vi "波形发生器模拟输出.vi"() -> ()   [LabVIEW 2017]
uses:
  <vilib>/DAQmx/write.llb/DAQmx Write (Analog Wfm 1Chan NSamp).vi
  <vilib>/DAQmx/create/channels.llb/DAQmx Create Channel (AO-Voltage-Basic).vi
  <vilib>/DAQmx/configure/timing.llb/DAQmx Timing (Sample Clock).vi
  <vilib>/DAQmx/miscellaneous.llb/DAQmx Fill In Error Info.vi
  <resource>/objmgr/daqmx.rc
panel:
  out "采集卡的采样率":dbl
  in  "Fs":dbl=1000.0 caption="采样率" format="%.2p"
  in  "#s":dbl=1000.0 caption="样本数"
  in  "噪声选择":i8(slide)
  out "最小值":dbl format="%#_3g"
  out "最大值":dbl format="%#_3g"
  out "频率":dbl
  in  "自定义波形":cluster{"输入坐标":bool, "手绘":bool, "输入公式":bool}
  in  "波形选择\n选择":bool
  in  "标准波形":i8(slide) scale=0.0..3.0
  out "自定义波形指示灯":bool
  out "标准波形指示灯":bool
  in  "相位":dbl
  in  "幅值":dbl
  in  "频率":dbl
  in  "停止":bool
  in  "噪声幅值":dbl=1.0 format="%.2p"
  in  "占空比":dbl=50.0 caption="占空比(%)" format="%0.2f"
  out "波形图":waveform(dbl)(graph)
  # "函 数 发 生 器"
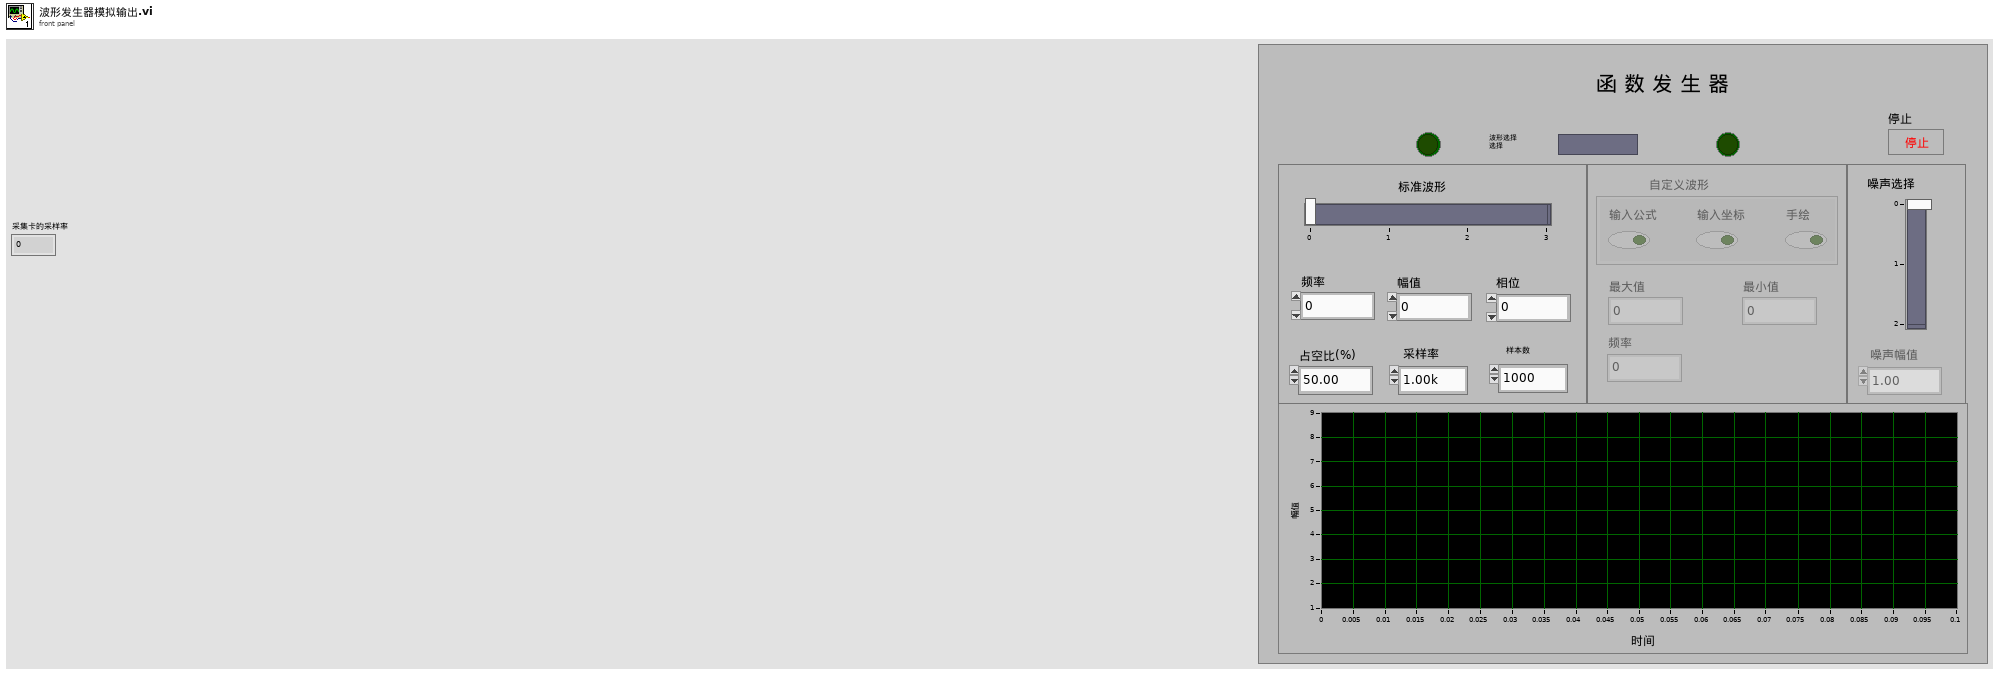
[diagram p1: front panel]
types:
  T1 = enum8{"Enabled", "Disabled", "Disabled and Grayed Out"}
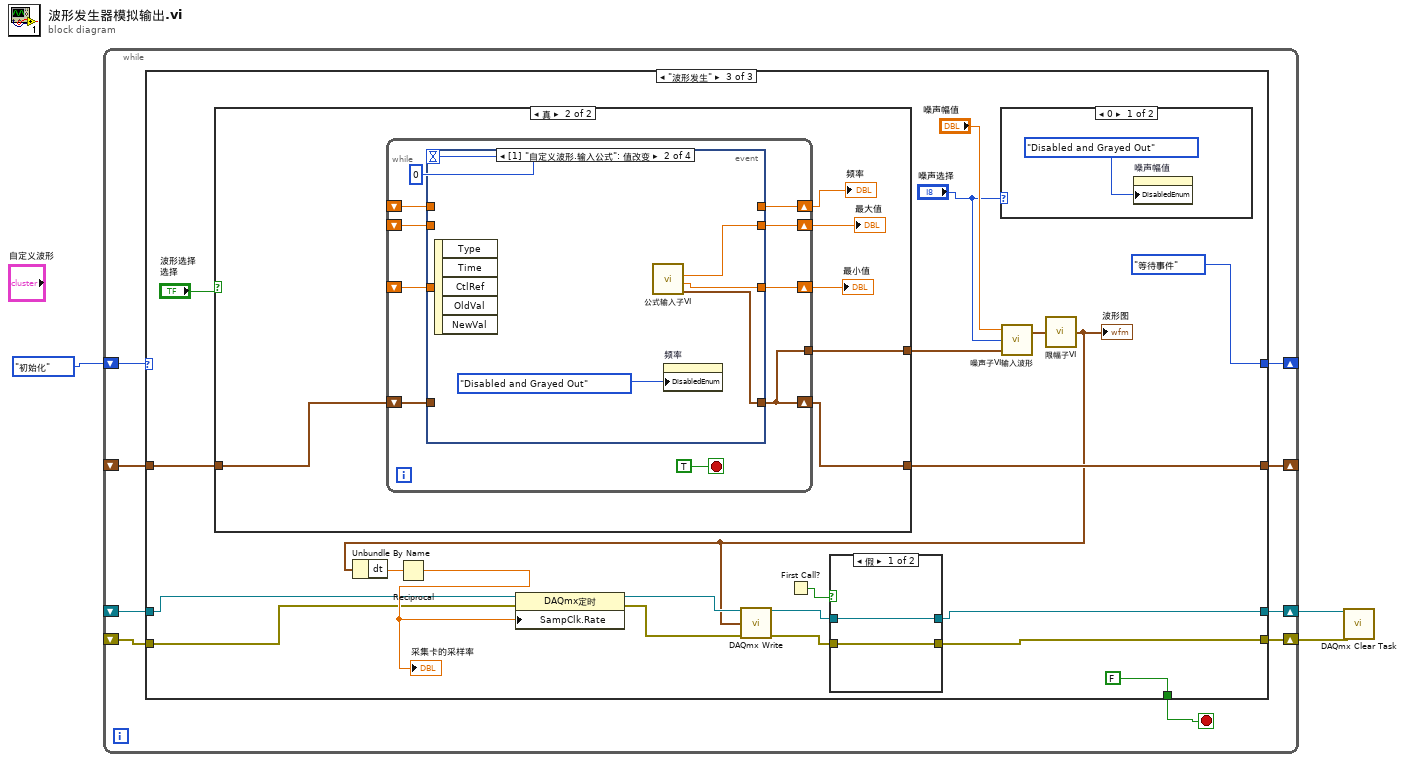
[diagram p0: block diagram]
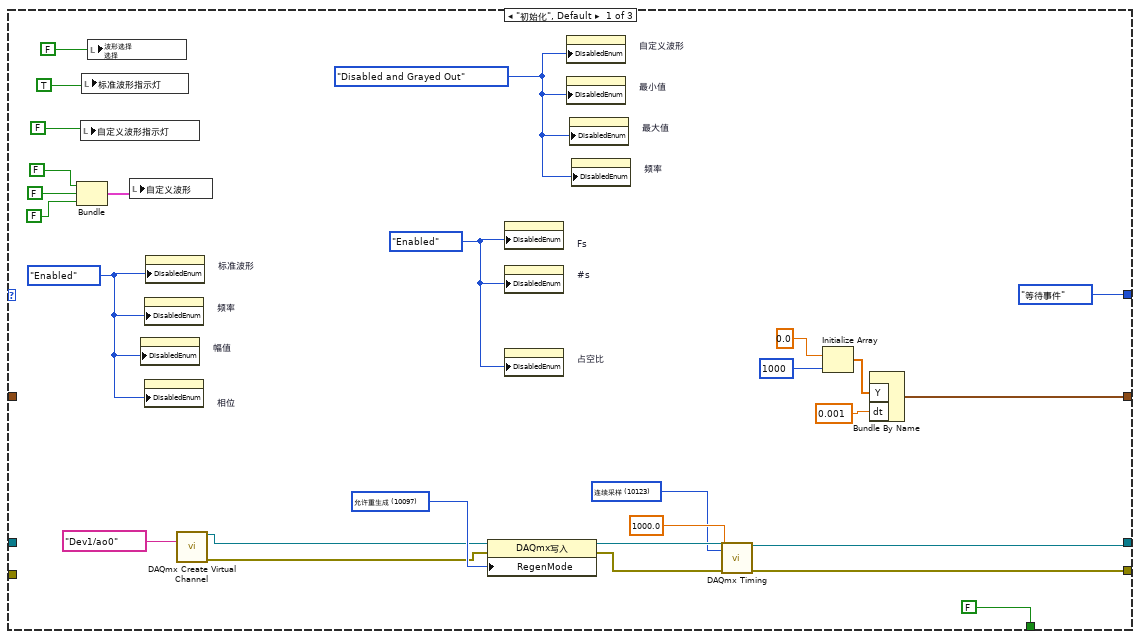
[diagram p2: hidden frame]
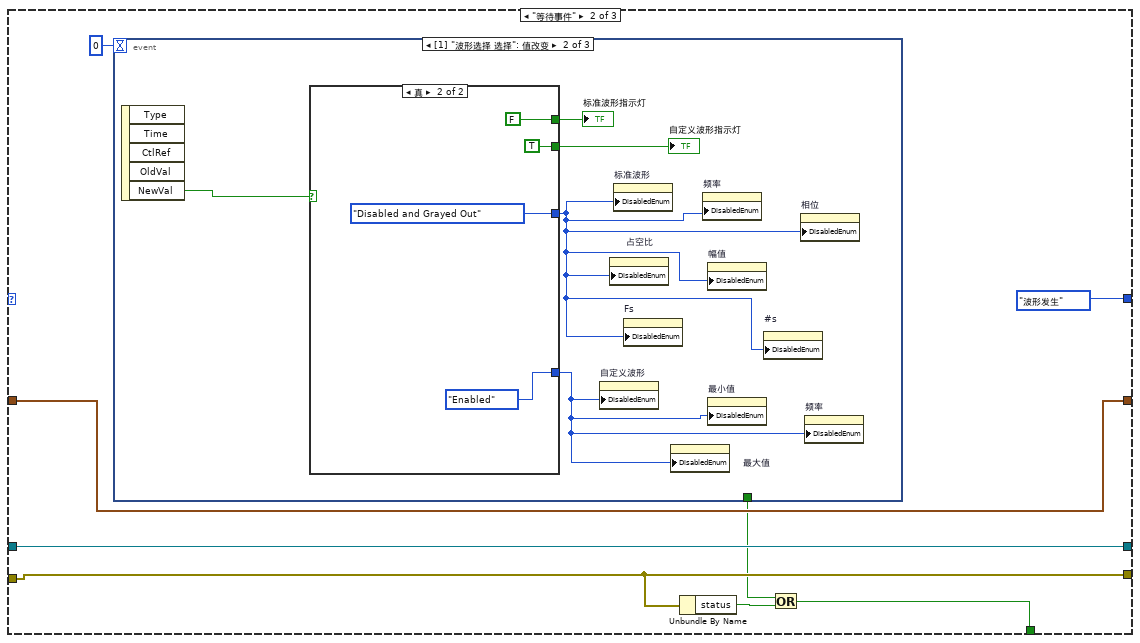
[diagram p3: hidden frame]
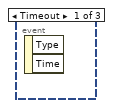
[diagram p4: hidden frame]
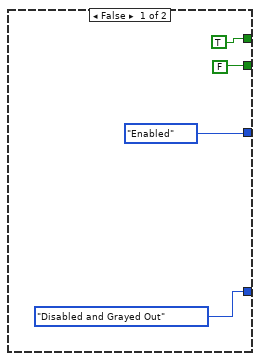
[diagram p5: hidden frame]
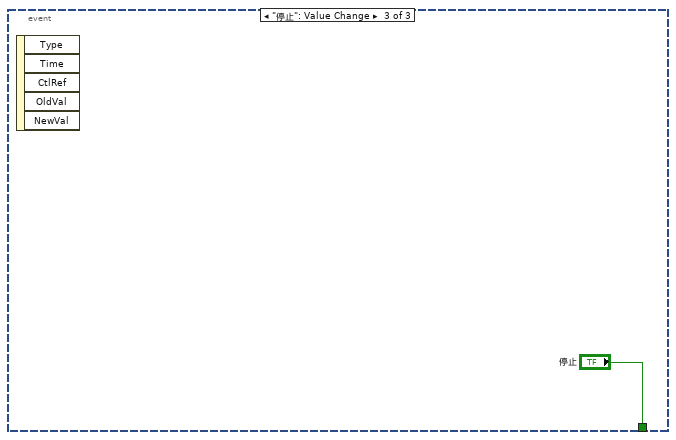
[diagram p6: hidden frame]
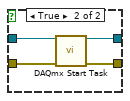
[diagram p7: hidden frame]
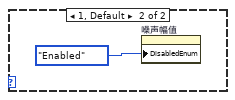
[diagram p8: hidden frame]
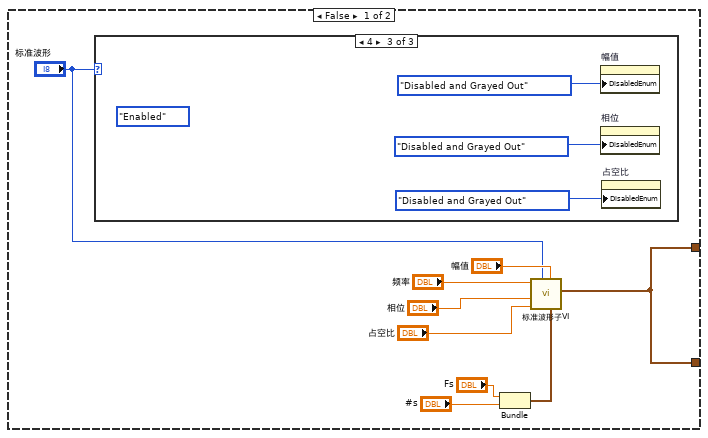
[diagram p9: hidden frame]
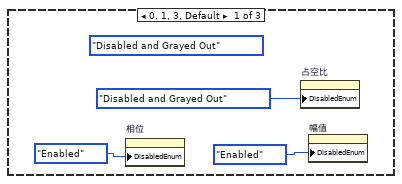
[diagram p10: hidden frame]
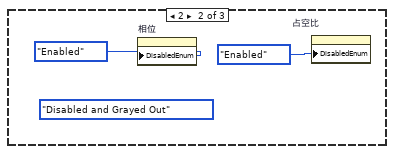
[diagram p11: hidden frame]
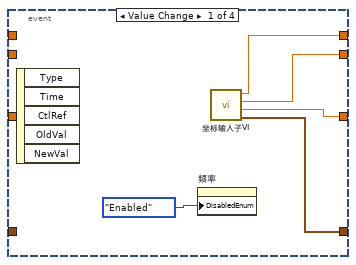
[diagram p12: hidden frame]
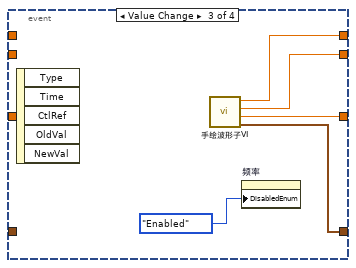
[diagram p13: hidden frame]
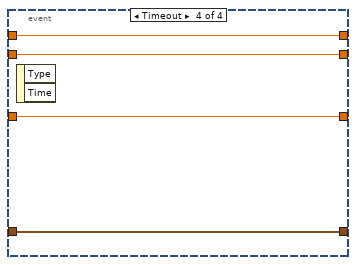
[diagram p14: hidden frame]
diagram:
  n1 = while {
    shift-right: [w11] -> _
    shift-left: enum16{"初始化", "等待事件", "波形发生", "停止"}."初始化" -> [w12]
    shift-right: [w9] -> _
    shift-left: _ -> [w10]
    shift-right: [w6] -> w2
    shift-left: _ -> [w8]
    shift-right: [w5] -> w1
    shift-left: _ -> [w7]
    stop <- w4 stop-if-true
    n2 = case shown="\"波形发生\"" w12 {
      tunnel: [enum16{"初始化", "等待事件", "波形发生", "停止"}."等待事件" enum16{"初始化", "等待事件", "波形发生", "停止"}."波形发生" enum16{"初始化", "等待事件", "波形发生"}."等待事件"] -> w11
      tunnel: w10 -> [_ w47 w76]
      tunnel: [w14 w47 w75] -> w9
      tunnel: w8 -> [_ w46 w66]
      tunnel: w7 -> [_ w44 w65]
      tunnel: [w24 w46 w64] -> w6
      tunnel: [w23 w44 w63] -> w5
      tunnel: [FALSE ("status") w41 FALSE ("status")] -> w4
      frame "初始化", Default {
        w29 = 10097 items=["允许重生成"=10097, "不允许重生成"=10158] ("RegenMode")
        w25 = 10123 items=["有限采样"=10178, "连续采样"=10123, "硬件定时单点"=12522] ("sample mode")
        w31 = T1."Enabled" ("禁用")
        w32 = T1."Enabled" ("禁用")
        w30 = T1."Disabled and Grayed Out" ("禁用")
        n3 = Bundle(FALSE, FALSE, FALSE) -> (w33:cluster{bool, bool, bool})  [unwired: 1 in]
        n4 = local write "自定义波形指示灯"(FALSE ("自定义波形")) -> ()
        n5 = local write "标准波形指示灯"(TRUE ("标准波形")) -> ()
        n6 = local write "波形选择\n选择"(FALSE ("波形选择")) -> ()
        n7 = local write "自定义波形"(w33) -> ()
        n8 = property on="幅值" class="DigNum (严格)"("DisabledEnum"=w32) -> ()  [unwired: 2 in, 2 out]
        n9 = property on="频率" class="DigNum (严格)"("DisabledEnum"=w32) -> ()  [unwired: 2 in, 2 out]
        n10 = property on="相位" class="DigNum (严格)"("DisabledEnum"=w32) -> ()  [unwired: 2 in, 2 out]
        n11 = property on="标准波形" class="Slide (严格)"("DisabledEnum"=w32) -> ()  [unwired: 2 in, 2 out]
        n12 = call-poly <vilib>:"DAQmx Create Virtual Channel.vi"("physical channels"=tag "Dev1/ao0") -> ("task out"=w21:refnum<k21>, "error out"=w20:errorcluster)  [unwired: 13 in]
        n13 = property class="DAQmx写入"(reference=w21, error in=w20, "RegenMode"=w29) -> (reference out=w27:refnum<k21>, error out=w28:errorcluster)
        n14 = property on="Fs" class="DigNum (严格)"("DisabledEnum"=w31) -> ()  [unwired: 2 in, 2 out]
        n15 = property on="#s" class="DigNum (严格)"("DisabledEnum"=w31) -> ()  [unwired: 2 in, 2 out]
        n16 = property on="占空比" class="DigNum (严格)"("DisabledEnum"=w31) -> ()  [unwired: 2 in, 2 out]
        n17 = property on="自定义波形" class="Clust (严格)"("DisabledEnum"=w30) -> ()  [unwired: 2 in, 2 out]
        n18 = property on="最小值" class="DigNum (严格)"("DisabledEnum"=w30) -> ()  [unwired: 2 in, 2 out]
        n19 = property on="最大值" class="DigNum (严格)"("DisabledEnum"=w30) -> ()  [unwired: 2 in, 2 out]
        n20 = property on="频率" class="DigNum (严格)"("DisabledEnum"=w30) -> ()  [unwired: 2 in, 2 out]
        n21 = call-poly <vilib>:"DAQmx Timing.vi"("task/channels in"=w27, "sample mode"=w25, "rate"=1000.0, "error in"=w28) -> ("task out"=w24:refnum<k21>, "error out"=w23:errorcluster)  [unwired: 10 in]
        n22 = Initialize Array(0.0 ("元素"), 1000 ("维数大小")) -> (w17:dbl[])
        n23 = Bundle By Name("Y"=w17, "dt"=0.001) -> (w14:waveform(dbl))  [unwired: 1 in]
      }
      frame "等待事件" {
        n24 = event shown="[1] \"波形选择 选择\": 值改变" {
          selector: _ -> [_ _ _]
          dyn-events: _ -> [_ _ _]
          timeout: 0 -> [_ _ _]
          tunnel: [_ _ "停止"] -> w43
          event Timeout {
            n25 = event-data() -> ()  [unwired: 1 in, 2 out]
          }
          event "波形选择\n选择": Value Change {
            n26 = event-data() -> ("NewVal"=w50:bool)  [unwired: 1 in, 4 out]
            n27 = case shown="真" w50 {
              tunnel: [TRUE FALSE] -> w52
              tunnel: [FALSE TRUE] -> w51
              tunnel: [T1."Enabled" ("禁用") T1."Disabled and Grayed Out" ("禁用")] -> w49
              tunnel: [T1."Disabled and Grayed Out" ("禁用") T1."Enabled" ("禁用")] -> w48
              frame False {
              }
              frame True {
              }
            }
            "标准波形指示灯" <- w52
            "自定义波形指示灯" <- w51
            n28 = property on="自定义波形" class="Clust (严格)"("DisabledEnum"=w48) -> ()  [unwired: 2 in, 2 out]
            n29 = property on="占空比" class="DigNum (严格)"("DisabledEnum"=w49) -> ()  [unwired: 2 in, 2 out]
            n30 = property on="标准波形" class="Slide (严格)"("DisabledEnum"=w49) -> ()  [unwired: 2 in, 2 out]
            n31 = property on="Fs" class="DigNum (严格)"("DisabledEnum"=w49) -> ()  [unwired: 2 in, 2 out]
            n32 = property on="最大值" class="DigNum (严格)"("DisabledEnum"=w48) -> ()  [unwired: 2 in, 2 out]
            n33 = property on="频率" class="DigNum (严格)"("DisabledEnum"=w49) -> ()  [unwired: 2 in, 2 out]
            n34 = property on="幅值" class="DigNum (严格)"("DisabledEnum"=w49) -> ()  [unwired: 2 in, 2 out]
            n35 = property on="最小值" class="DigNum (严格)"("DisabledEnum"=w48) -> ()  [unwired: 2 in, 2 out]
            n36 = property on="#s" class="DigNum (严格)"("DisabledEnum"=w49) -> ()  [unwired: 2 in, 2 out]
            n37 = property on="相位" class="DigNum (严格)"("DisabledEnum"=w49) -> ()  [unwired: 2 in, 2 out]
            n38 = property on="频率" class="DigNum (严格)"("DisabledEnum"=w48) -> ()  [unwired: 2 in, 2 out]
          }
          event "停止": Value Change {
            n39 = event-data() -> ()  [unwired: 1 in, 5 out]
          }
        }
        n40 = Unbundle By Name(w44) -> ("status"=w42:bool)
        n41 = Or(x=w43, y=w42) -> (x .or. y?=w41:bool)
      }
      frame "波形发生" {
        n42 = case shown="真" "波形选择\n选择" {
          tunnel: [w93 w113] -> w80
          tunnel: w76 -> [_ w110]
          tunnel: [w93 w109] -> w75
          frame False {
            n43 = case shown="4" "标准波形" {
              frame 0, 1, 3, Default {
                (unwired) T1."Disabled and Grayed Out" ("禁用")
                n44 = property on="相位" class="DigNum (严格)"("DisabledEnum"=T1."Enabled" ("禁用")) -> ()  [unwired: 2 in, 2 out]
                n45 = property on="占空比" class="DigNum (严格)"("DisabledEnum"=T1."Disabled and Grayed Out" ("禁用")) -> ()  [unwired: 2 in, 2 out]
                n46 = property on="幅值" class="DigNum (严格)"("DisabledEnum"=T1."Enabled" ("禁用")) -> ()  [unwired: 2 in, 2 out]
              }
              frame 2 {
                (unwired) T1."Disabled and Grayed Out" ("禁用")
                n47 = property on="相位" class="DigNum (严格)"("DisabledEnum"=T1."Enabled" ("禁用")) -> ()  [unwired: 2 in, 2 out]
                n48 = property on="占空比" class="DigNum (严格)"("DisabledEnum"=T1."Enabled" ("禁用")) -> ()  [unwired: 2 in, 2 out]
              }
              frame 4 {
                (unwired) T1."Enabled" ("禁用")
                n49 = property on="幅值" class="DigNum (严格)"("DisabledEnum"=T1."Disabled and Grayed Out" ("禁用")) -> ()  [unwired: 2 in, 2 out]
                n50 = property on="相位" class="DigNum (严格)"("DisabledEnum"=T1."Disabled and Grayed Out" ("禁用")) -> ()  [unwired: 2 in, 2 out]
                n51 = property on="占空比" class="DigNum (严格)"("DisabledEnum"=T1."Disabled and Grayed Out" ("禁用")) -> ()  [unwired: 2 in, 2 out]
              }
            }
            n52 = Bundle("Fs"="Fs", "#s"="#s") -> (w94:cluster{"Fs":dbl, "#s":dbl})  [unwired: 1 in]
            n53 = call "标准波形子VI.vi"("采样信息"=w94, "幅值"="幅值", "波形选择"="标准波形", "方波占空比"="占空比", "相位"="相位", "频率"="频率") -> ("波形图"=w93:waveform(dbl))  [unwired: 5 in]
          }
          frame True {
            n54 = while {
              tunnel: [w121] -> w113
              shift-right: [w121] -> w109
              shift-left: w110 -> [w120]
              shift-right: [w119] -> w108
              shift-left: _ -> [w118]
              shift-right: [w117] -> w112
              shift-left: _ -> [w115]
              shift-right: [w116] -> w111
              shift-left: _ -> [w114]
              stop <- TRUE stop-if-true
              n55 = event shown="[1] \"自定义波形.输入公式\": 值改变" {
                selector: _ -> [_ _ _ _]
                dyn-events: _ -> [_ _ _ _]
                timeout: 0 -> [_ _ _ _]
                tunnel: [w125 w130 w134 w141] -> w121
                tunnel: w120 -> [_ _ _ w141]
                tunnel: [w128 _ w137 w140] -> w119
                tunnel: w118 -> [_ _ _ w140]
                tunnel: [w127 w132 w136 w139] -> w117
                tunnel: [w126 w131 w135 w138] -> w116
                tunnel: w115 -> [_ _ _ w139]
                tunnel: w114 -> [_ _ _ w138]
                event "自定义波形.输入坐标": Value Change {
                  n56 = event-data() -> ()  [unwired: 1 in, 5 out]
                  n57 = property on="频率" class="DigNum (严格)"("DisabledEnum"=T1."Enabled" ("禁用")) -> ()  [unwired: 2 in, 2 out]
                  n58 = call "坐标输入子VI.vi"() -> ("生成的波形"=w125:waveform(dbl), "最小值"=w126:dbl, "最大值"=w127:dbl, "频率"=w128:dbl)  [unwired: 4 in]
                }
                event "自定义波形.输入公式": Value Change {
                  n59 = event-data() -> ()  [unwired: 1 in, 5 out]
                  n60 = call "公式输入子VI .vi"() -> ("生成的波形"=w130:waveform(dbl), "最小值"=w131:dbl, "最大值"=w132:dbl)  [unwired: 5 in]
                  n61 = property on="频率" class="DigNum (严格)"("DisabledEnum"=T1."Disabled and Grayed Out" ("禁用")) -> ()  [unwired: 2 in, 2 out]
                }
                event "自定义波形.手绘": Value Change {
                  n62 = event-data() -> ()  [unwired: 1 in, 5 out]
                  n63 = call "手绘波形子VI.vi"() -> ("输出的波形"=w134:waveform(dbl), "最小值"=w135:dbl, "最大值"=w136:dbl, "频率"=w137:dbl)  [unwired: 4 in]
                  n64 = property on="频率" class="DigNum (严格)"("DisabledEnum"=T1."Enabled" ("禁用")) -> ()  [unwired: 2 in, 2 out]
                }
                event Timeout {
                  n65 = event-data() -> ()  [unwired: 1 in, 2 out]
                }
              }
            }
            "频率" <- w108
            "最大值" <- w112
            "最小值" <- w111
          }
        }
        n66 = First Call?() -> (First Call?: T/F=w71:bool)
        n67 = case shown="0" "噪声选择" {
          frame 0 {
            n68 = property on="噪声幅值" class="DigNum (严格)"("DisabledEnum"=T1."Disabled and Grayed Out" ("禁用")) -> ()  [unwired: 2 in, 2 out]
          }
          frame 1, Default {
            n69 = property on="噪声幅值" class="DigNum (严格)"("DisabledEnum"=T1."Enabled" ("禁用")) -> ()  [unwired: 2 in, 2 out]
          }
        }
        n70 = call "噪声子VI输入波形.vi"("输入波形"=w80, "噪声选择"="噪声选择", "幅值"="噪声幅值") -> ("波形图"=w79:waveform(dbl))  [unwired: 1 in]
        n71 = call "限幅子VI.vi"("波形"=w79) -> ("输出波形"=w68:waveform(dbl))
        "波形图" <- w68
        n72 = Unbundle By Name(w68) -> ("dt"=w67:dbl)
        n73 = Reciprocal(x=w67) -> (1/x=w72:dbl)
        "采集卡的采样率" <- w72
        n74 = property class="DAQmx定时"(reference=w66, error in=w65, "SampClk.Rate"=w72) -> (reference out=w74:refnum<k21>, error out=w73:errorcluster)
        n75 = call-poly <vilib>:"DAQmx Write.vi"("task/channels in"=w74, "data"=w68, "error in"=w73) -> ("task out"=w70:refnum<k21>, "error out"=w69:errorcluster)  [unwired: 10 in, 1 out]
        n76 = case shown="假" w71 {
          tunnel: w70 -> [w84 w88]
          tunnel: w69 -> [w83 w87]
          tunnel: [w84 w86] -> w64
          tunnel: [w83 w85] -> w63
          frame False {
          }
          frame True {
            n77 = call <vilib>:"DAQmx Start Task.vi"("task/channels in"=w88, "error in"=w87) -> ("task out"=w86:refnum<k21>, "error out"=w85:errorcluster)  [unwired: 12 in]
          }
        }
      }
    }
  }
  n78 = call <vilib>:"DAQmx Clear Task.vi"("task in"=w2, "error in"=w1) -> ()  [unwired: 13 in, 1 out]
